vi "trace_toLVBuffer_spectrum.vi"(0 "reference":refnum<class "OSA.lvclass">, 2 "idx latest":bool, 3 "trace idx spectrum":u32, 5 "error in (no error)":errorcluster) -> (14 "duplicate reference":refnum<class "OSA.lvclass">, 16 "trace length":u32, 19 "error out":errorcluster)   [LabVIEW 2010, in "OSA.lvclass"]
doc: "Reads data from trace buffer and updates labview allocated buffer interferogram Y array, X is equidistant and only x min and max are retrieved. \n\nX: optical path length (cm)\nY: ADC value"
uses:
  OSA.lvclass
  typeDef/trace_properties_ui.ctl
  typeDef/trace_properties_double.ctl
  typeDef/acq_dataType.ctl
  typeDef/xVal_option.ctl
  FTSLib.dll
  OSA20X_misc.lvlib
panel:
  in  "property double":T1=enum."x_max"
  in  "property":T2=enum."interferogramProperty"
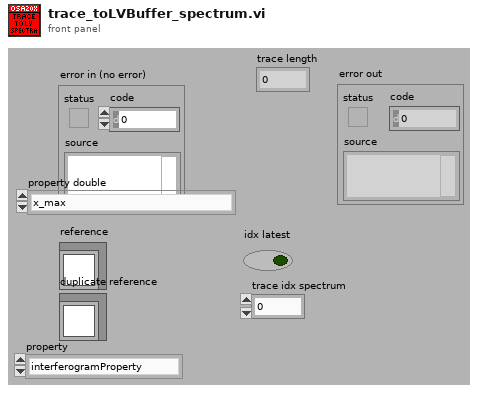
[diagram p1: front panel]
types:
  T1 = typedef "OSA.lvclass/trace_properties_double.ctl" = enum16{"x_minWnr", "x_maxWnr", "x_min", "x_max", "y_min", "y_max", "resolution", "referenceWavelength_nm_vac", "samplingDistance_cm_vac", "zeroFillFactor", "air_temp", "air_press", "air_relHum", "minOPD_cm", "maxOPD_cm", "interferogramOffset", "apodizationPowerCompensation", "integrationTime_ms", "gainLevel", "all_doubleProperties"}
  T2 = typedef "OSA.lvclass/trace_properties_ui.ctl" = enum16{"length", "type", "acquisitionMode", "xValueFormat", "date", "time", "averageNum", "smoothType", "igramSmoothType", "phaseCorrection", "apodisation", "__allocatedLengthI", "__allocatedLengthx", "adcBits", "sensitivityMode", "resolutionMode", "rollingAverage", "samplesPerReference", "air_measureOption", "interferogramProperty", "all_uiProperties"}
  T3 = typedef "OSA.lvclass/acq_dataType.ctl" = enum16{"none", "interferogram", "spectrum"}
  T4 = enum16{"get", "init", "set interferogram", "set spectrum", "cleanUp"}
  T5 = typedef "OSA.lvclass/xVal_option.ctl" = enum16{"MIN_MAX", "ARRAY"}
  T6 = typedef "OSA.lvclass/ObjectAttributes.ctl" = cluster{"Stop":bool, "dataType":T3, "spectrometerIdx":u16, "buffer size interferogram":i32, "interferogram":cluster{"new":bool, "plot_x_ min":sgl, "plot_x_max":sgl, "plot_y_min":sgl, "plot_y_max":sgl, "Graph Intrfrgrm":T7, "timeStamp":u32, "signal (%)":dbl, "traces":cluster{"idx":u32, "broadBand":bool, "monoChromatic":bool, "peakToPeakSignal":dbl, "peakToPeakPos":dbl}[], "traces idx last":i32}, "spectrum":cluster{"new":bool, "plot_x_min":sgl, "plot_x_max":sgl, "plot_unit_x":T8, "plot_unit_y":T9, "plot_y_min":sgl, "plot_y_max":sgl, "Graph Spectrum":T7, "timeStamp":u32, "X_VAL_OPTIONS":enum16{"MIN_MAX", "ARRAY"}, "traces":cluster{"idx":u32}[], "traces idx last":i32}, "Thorlabs_OSA_64.lvclass:queue_action.ctlqueue ref":refnum<queue>, "action":T10, "plot zoom step":dbl, "buffer semaphore":T11, "acq stopped":bool, "dataType active":T3, "temperature (degr C)":sgl, "pressure (hPa)":sgl, "rel humidity (%)":sgl, "settings":cluster{"resolution":T12, "sensitivity":T13, "Average":bool, "average nr":u32, "apodisation":T14, "acq delay (ms)":u32, "airMesure":T15, "wmtr on":bool, "intfgrm_smooth_width":u16, "intfgrm_smooth_nrOfPasses":u16, "intfgrm_smooth":T16, "phaseCorrection":T17, "zeroFill":u8, "spectr_smooth":T16, "spectr_smooth_width":u16, "spectr_smooth_nrOfPasses":u16, "resolution (/cm)":sgl, "REF wavelength, (nm)":dbl, "gain_idx":u16, "gainAuto":bool, "gain_relative":dbl, "PD sensitivity mode":T18, "PD senseMode implemented":bool, "SensorTemperature implemented":bool, "SensorPressure implemented":bool, "SensorHumidity implemented":bool}, "peaks position":sgl[], "peaks width":sgl[], "peaks height":sgl[], "peaks max nr":u32, "peaks latest nr":i32, "peaks new":bool, "power":dbl, "power new":bool, "path":string, "wavelength (WNr)":dbl, "wavelength new":bool, "buffer size spectrum":i32, "status":string, "VI reference":refnum<vi>, "funcPointer":u64, "libraryPointer":u64, "singleAcquisition":bool, "coherenceLength (cm)":dbl, "coherenceLength new":bool, "spectrometer model":string, "spectrometer serial nr":string, "peaks thld left":sgl[], "peaks thld right":sgl[], "coherenceLength error (cm)":dbl, "ADC bits":u16, "peaks position centroid":sgl[], "peaks height centroid":sgl[], "OSA series":T19, "channel index spectra":u16, "channel index interferogram":u16}
  T7 = typedef "OSA.lvclass/graph_intensity.ctl" = refnum<vi>
  T8 = typedef "OSA.lvclass/spectrum_x_unit.ctl" = enum16{"wavenr/cm", "THz", "eV", "nm_air", "nm_vac"}
  T9 = typedef "OSA.lvclass/y_unit.ctl" = enum16{"ADC counts", "dBm pwr absolute", "dBm pwr density", "mW pwr absolute", "mW pwr density"}
  T10 = typedef "OSA.lvclass/queue_action.ctl" = enum16{"none", "stop", "GUI_plotInterferogram", "GUI_plotSpectrum", "GUI_plotInterferogramRescale", "GUI_plotSpectrumRescale", "GUI_plotInterferogramReset", "GUI_plotSpectrumReset", "GUI_plotInterferogramAutoScaleY", "GUI_plotSpectrumAutoScaleY", "GUI_plotInterferogramZoomOut", "GUI_plotSpectrumZoomOut", "GUI_plotInterferogramPane", "GUI_plotSpectrumPane", "GUI_plotInterferogramZoomMouse", "GUI_plotSpectrumZoomMouse", "ENVIRONMENT temperature", "ENVIRONMENT pressure", "MODE_resolution set", "MODE_resolution get", "MODE_sensitivity set", "MODE_sensitivity get", "MODE_PDTemperature set", "MODE_PDTemperature get", "REBOOT/RESET firmware", "ACQASYNC_acquireSingleSpectrum", "ACQASYNC_continuous start", "ACQASYNC_continuous stop\n", "ACQASYNC_get last interferogram", "ACQASYNC_get last spectrum", "ACQASYNC_get last waveNr", "ACQOPT_interferogram smoothing set", "ACQOPT_interferogram smoothing get", "ACQOPT_spectrum smoothing set", "ACQOPT_spectrum smoothing get", "ACQOPT_apodisation type set", "ACQOPT_apodisation type get", "ACQOPT_phase correction type set", "ACQOPT_phase correction type get", "ACQOPT_acqIntervall_set", "ACQOPT_acqIntervall_get", "ACQOPT_average spectrum set", "ACQOPT_average spectrum get", "ACQOPT_rolling average set", "ACQOPT_rolling average get", "ACQOPT_zero fill factor set", "ACQOPT_zero fill factor get", "ACQOPT_cycle counting set", "ACQOPT_cycle counting get", "ACQOPT_air measure option set", "ACQOPT_air measure option get", "ACQOPT_gainLevel auto get", "ACQOPT_gainLevel auto set", "ACQOPT_gainLevel get", "ACQOPT_gainLevel set", "ACQOPT_getAll", "INSTRUMENT_PROPERTY_range_WaveNr_min", "INSTRUMENT_PROPERTY_range_WaveNr_max", "INSTRUMENT_PROPERTY_reference_wavelength_cm^-1", "INSTRUMENT_PROPERTY_samplesPerRefPeriod", "INSTRUMENT_PROPERTY_resolution_waveNrPercm", "INSTRUMENT_PROPERTY_availableGainLevels", "INSTRUMENT_PROPERTY_status", "CONVERT", "ANALYSE_POWER", "ANALYSE_PEAKS", "ANALYSE_WAVELENGTH", "ANALYSE_SPECTRUM", "ANALYSE_INTERFEROGRAM", "ANALYSE_COHERENCE_LENGTH", "MATH", "MATH_power", "MATH_peaks", "FILE", "miscellaneous"}
  T11 = typedef "Semaphore RefNum" = refnum<k1>
  T12 = typedef "OSA.lvclass/resolution.ctl" = enum16{"low", "high"}
  T13 = typedef "OSA.lvclass/sensitivityMode.ctl" = enum16{"low", "low medium", "high medium", "high"}
  T14 = typedef "OSA.lvclass/apodisation.ctl" = enum16{"NONE", "NORTON_BEER_WEAK", "NORTON_BEER_MEDIUM", "NORTON_BEER_STRONG", "TRIANGULAR", "COSINE", "HANN", "HAMMING", "BLACKMANHARRIS3", "BLACKMANHARRIS4", "GAUSSIAN"}
  T15 = typedef "OSA.lvclass/airMeasure.ctl" = enum16{"TEMPERATURE", "PRESSURE"}
  T16 = typedef "OSA.lvclass/smoothing.ctl" = enum16{"NONE", "BINOMIAL", "SAVITSKY_GOLAY", "FOURIER", "MOVING_AVERAGE", "GAUSSIAN"}
  T17 = typedef "OSA.lvclass/phaseCorrection.ctl" = enum16{"NONE", "MERTZ", "FORMAN", "MERTZ_FILE", "FORMAN_FILE", "FUTURE COMP."}
  T18 = typedef "OSA.lvclass/PDTemperatureMode.ctl" = enum16{"cool: better sensitivity/noise floor", "warm: extended wl range"}
  T19 = typedef "OSA.lvclass/OSA_series.ctl" = enum16{"OSA200", "OSA300", "UNKNOWN"}
  T20 = typedef "OSA20X.lvclass/xVal_option.ctl" = enum16{"MIN_MAX", "ARRAY"}
  T21 = cluster{"length":u32, "X min":sgl, "X max":sgl, "X_VAL_OPTIONS":T20}
  T22 = cluster{"idx":u32, "broadBand":bool, "monoChromatic":bool, "peakToPeakSignal":dbl, "peakToPeakPos":dbl}[]
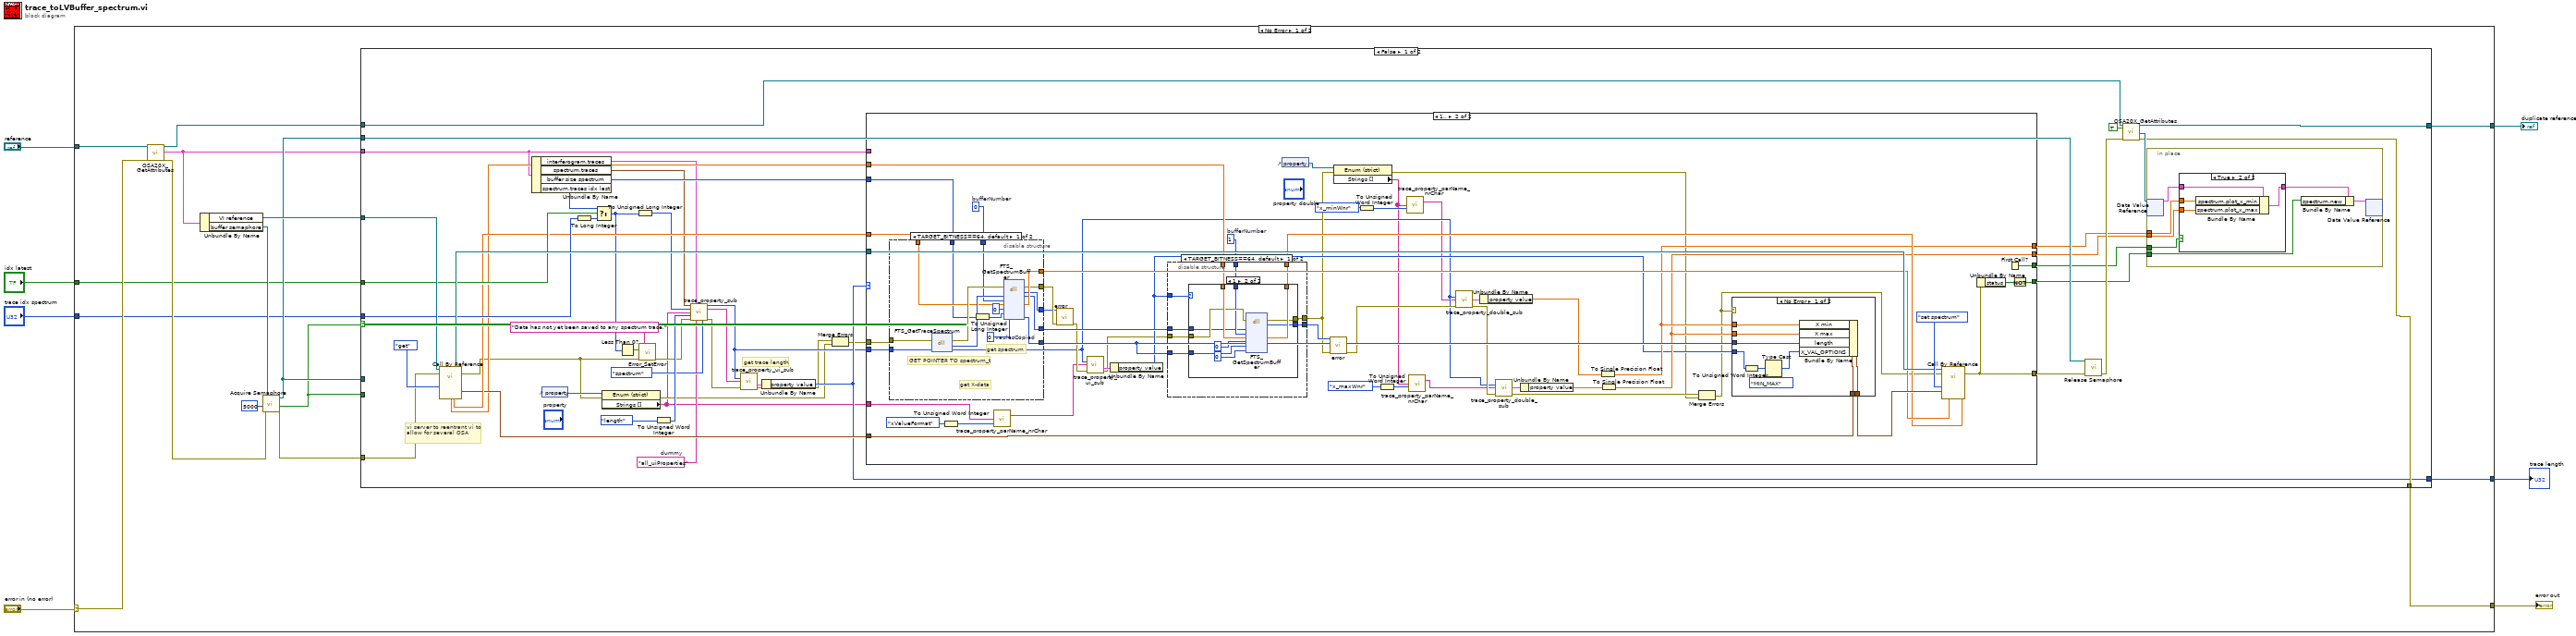
[diagram p0: block diagram]
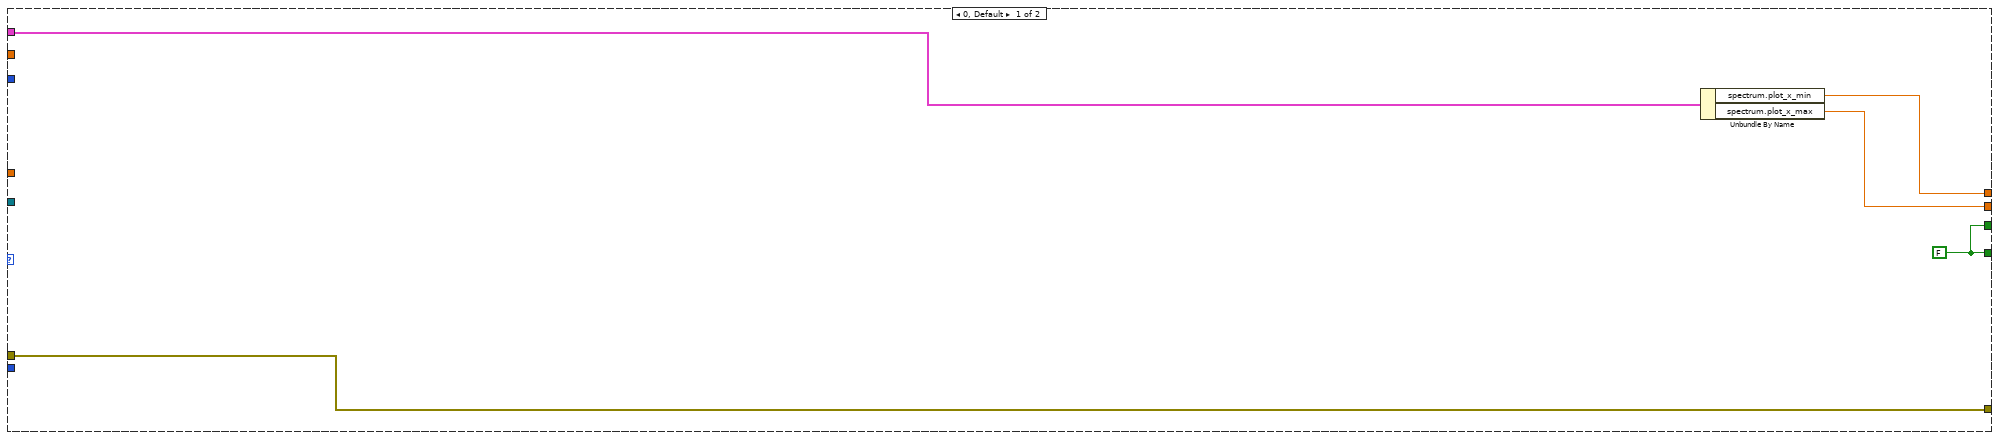
[diagram p2: hidden frame]
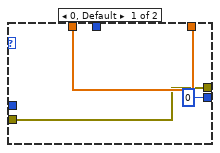
[diagram p3: hidden frame]
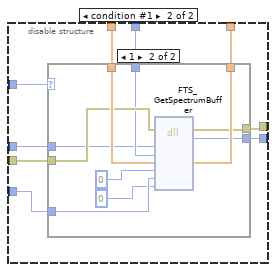
[diagram p4: hidden frame]
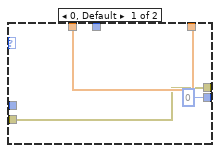
[diagram p5: hidden frame]
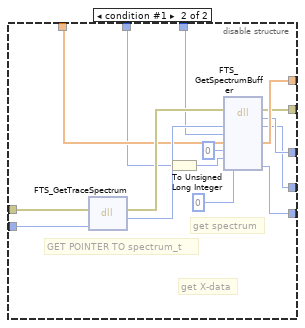
[diagram p7: hidden frame]
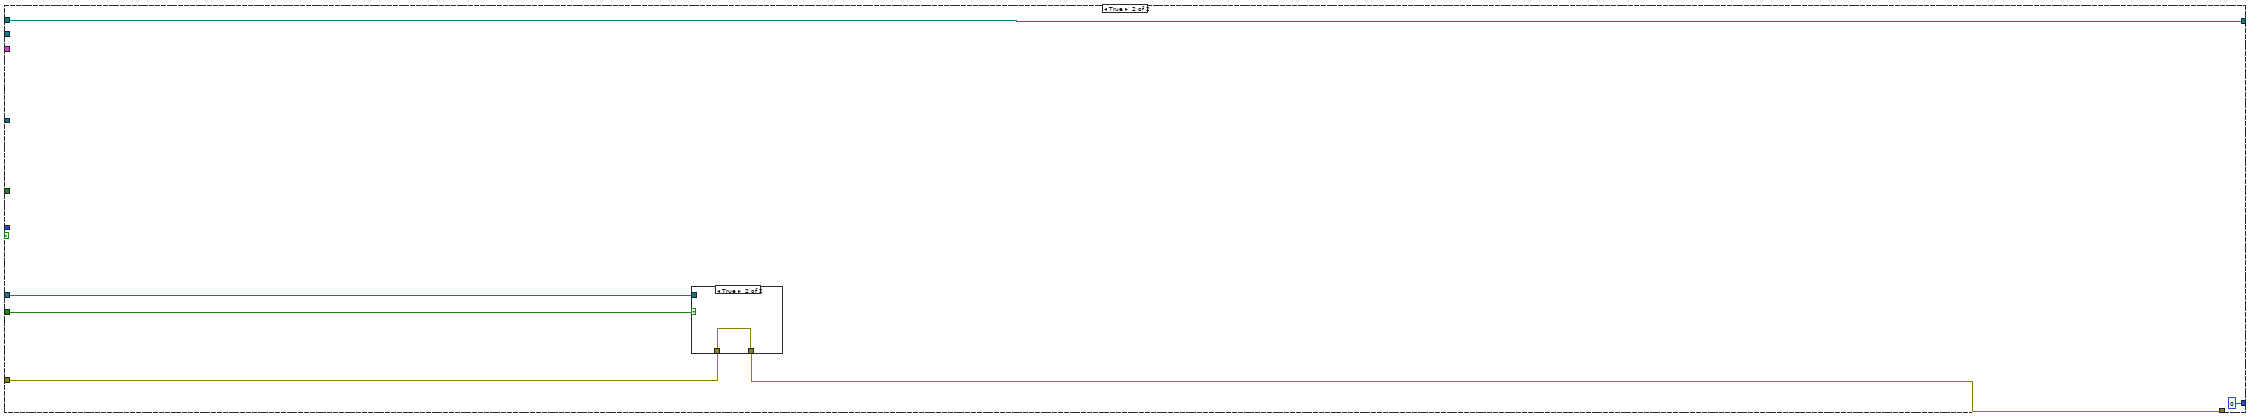
[diagram p9: hidden frame]
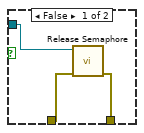
[diagram p10: hidden frame]
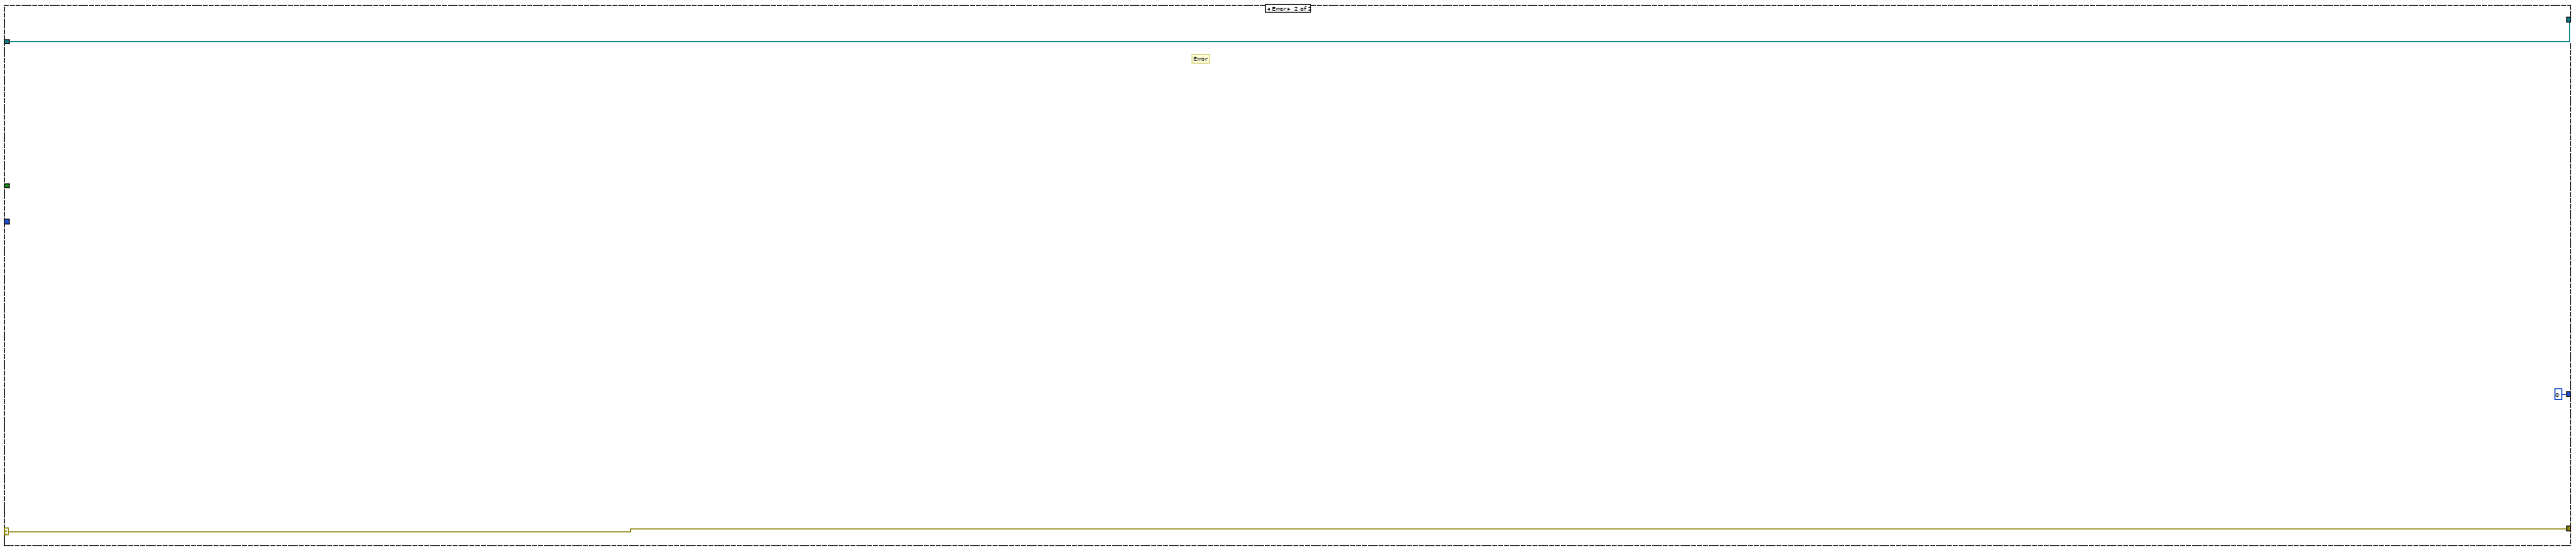
[diagram p11: hidden frame]
diagram:
  n1 = case shown="No Error" "error in (no error)" {
    selector: "error in (no error)" -> [w22 w234]
    tunnel: [w21 w234] -> w6
    tunnel: "reference" -> [w23 w233]
    tunnel: [w20 w233] -> w4
    tunnel: "idx latest" -> [w11 _]
    tunnel: "trace idx spectrum" -> [w10 _]
    tunnel: [w9 u32 0 ("property value")] -> w1
    frame No Error {
      n2 = call "OSA20X_GetAttributes.vi"("reference in"=w23, "error in (no error)"=w22) -> ("reference out"=w14:refnum<class "OSA.lvclass">, "Data"=w12:T6, "error out"=w18:errorcluster)  [unwired: 14 in, 1 out]
      n3 = Unbundle By Name(w12) -> ("VI reference"=w15:refnum<vi>, "buffer semaphore"=w19:T11)
      n4 = call <vilib>:"Acquire Semaphore.vi"("error in (no error)"=w18, "ms timeout (-1)"=5000, "semaphore"=w19) -> ("error out"=w16:errorcluster, "timed out"=w8:bool, "semaphore out"=w13:T11)  [unwired: 2 in]
      n5 = case shown="False" w8 {
        tunnel: w12 -> [w47 _]
        tunnel: w16 -> [w66 w224]
        tunnel: [w51 w223] -> w21
        tunnel: [w52 w227] -> w20
        tunnel: w13 -> [w68 _]
        tunnel: w15 -> [w65 _]
        tunnel: w14 -> [w25 w227]
        tunnel: w8 -> [_ w226]
        tunnel: w13 -> [_ w225]
        tunnel: w11 -> [w61 _]
        tunnel: w10 -> [w59 _]
        tunnel: [w30 u32 0 ("property value")] -> w9
        frame False {
          w32 = "all_uiProperties"  # dummy
          # "get trace length"
          # "vi server to reentrant vi to \nallow for several OSA"
          n6 = call-by-ref "?"(reference=w65, error in=w66, "action"=T4."get") -> (reference out=w64:refnum<vi>, error out=w43:errorcluster, "spectrum X"=w50:sgl[], "spectrum Y"=w54:sgl[], "spectrum property"=w53:T21)  [unwired: 14 in, 2 out]
          n7 = Unbundle By Name(w47) -> ("interferogram.traces"=w39:T22, "spectrum.traces"=w40:cluster{"idx":u32}[], "buffer size spectrum"=w55:i32, "spectrum.traces idx last"=w60:i32)
          n8 = control-ref of="property"() -> (w44:refnum<vi>)
          n9 = To Long Integer(number=w59) -> (32bit integer=w58:i32)
          n10 = Select(t=w60, s=w61, f=w58) -> (s? t:f=w41:i32)
          n11 = property class="Enum (strict)"(reference=w44, error in=w43) -> (error out=w27:errorcluster, "Strings []"=w24:string[])  [unwired: 1 out]
          n12 = Less Than 0?(x=w41) -> (x < 0?=w57:bool)
          n13 = To Unsigned Long Integer(number=w41) -> (unsigned 32bit integer=w38:u32)
          n14 = call "Error_SetError.vi"("error in"=w43, "status (true)"=w57, "source(\"\")"="Data has not yet been saved to any spectrum trace." ("source(\"\")")) -> ("error out"=w35:errorcluster)  [unwired: 4 in]
          n15 = To Unsigned Word Integer(number=trace_properties_ui."length" ("property")) -> (unsigned 16bit integer=w37:u16)
          n16 = call "trace_property_sub.vi"("traces_spectrum"=w40, "traces_interferogram"=w39, "trace idx"=w38, "Strings enum"=w24, "Value enum"=w37, "error in (no error)"=w35, "all string"=w32, "dataType"=acq_dataType."spectrum") -> ("global trace idx"=w29:u32, "parameter names"=w36:string[], "error out"=w34:errorcluster)  [unwired: 4 in, 1 out]
          n17 = call "trace_property_ui_sub.vi"("trace idx global"=w29, "properties ui"=w36, "error in (no error)"=w34) -> ("property"=w31:cluster{"property":string, "property value":u32}, "error out"=w28:errorcluster)  [unwired: 10 in, 1 out]
          n18 = Unbundle By Name(w31) -> ("property value"=w30:u32)
          n19 = Merge Errors(w28, w27) -> (w26:errorcluster)
          n20 = case shown="1.." w30 {
            tunnel: [w72 w105] -> w69
            tunnel: w64 -> [_ w124]
            tunnel: w55 -> [_ w123]
            tunnel: w54 -> [_ w122]
            tunnel: w53 -> [_ w121]
            tunnel: w29 -> [_ w88]
            tunnel: w26 -> [w72 w117]
            tunnel: w50 -> [_ w114]
            tunnel: [w74 w107] -> w49
            tunnel: [w73 w106] -> w48
            tunnel: w47 -> [w75 _]
            tunnel: [w71 w103] -> w46
            tunnel: [w71 w102] -> w45
            tunnel: w24 -> [_ w83]
            frame 0, Default {
              w71 = FALSE ("interferogram.new")
              n21 = Unbundle By Name(w75) -> ("spectrum.plot_x_min"=w74:sgl, "spectrum.plot_x_max"=w73:sgl)
            }
            frame 1.. {
              w112 = 1  # bufferNumber
              w119 = 0  # bufferNumber
              n22 = disable-structure shown="TARGET_BITNESS==64, default" {
                disable-tunnel: w117 -> [w193 w201]
                disable-tunnel: w88 -> [w194 w200]
                disable-tunnel: w122 -> [w190 w204]
                disable-tunnel: w123 -> [w188 w203]
                disable-tunnel: [w186 w199] -> w111
                disable-tunnel: [w185 w198] -> w118
                disable-tunnel: w119 -> [w183 w202]
                disable-tunnel: [w182 w197] -> w116
                disable-tunnel: [w181 w196] -> w115
                disable-tunnel: [w180 w195] -> w113
                frame condition #0 (active) {
                  w187 = u32 0  # vaulesCopied
                  # "get X-data"
                  # "get spectrum"
                  # "GET POINTER TO spectrum_t"
                  n23 = dll-call lib="FTSLib.dll" fn="FTS_GetTraceSpectrum"(error in=w193, "traceIdx"=w194) -> (error out=w192:errorcluster, "spectrum_t_pointer"=w191:u64)  [unwired: 3 in, 1 out]
                  n24 = To Unsigned Long Integer(number=w188) -> (unsigned 32bit integer=w184:u32)
                  n25 = dll-call lib="FTSLib.dll" fn="FTS_GetSpectrumBuffer"(error in=w192, "source"=w191, "bufferNumber"=w183, "destination"=w190, "startIndex"=u32 0, "length"=w184, "vaulesCopied"=w187) -> (error out=w182:errorcluster, "return type"=w181:i32, "source"=w180:u64, "destination"=w185:sgl[], "vaulesCopied"=w186:u32)  [unwired: 5 in, 1 out]
                }
                frame condition #1 {
                  # "get X-data"
                  # "get spectrum"
                  # "GET POINTER TO spectrum_t"
                  n26 = dll-call lib="FTSLib.dll" fn="FTS_GetTraceSpectrum"(error in=w201, "traceIdx"=w200) -> (error out=w209:errorcluster, "spectrum_t_pointer"=w208:u32)  [unwired: 3 in, 1 out]
                  n27 = To Unsigned Long Integer(number=w203) -> (unsigned 32bit integer=w205:u32)
                  n28 = dll-call lib="FTSLib.dll" fn="FTS_GetSpectrumBuffer"(error in=w209, "source"=w208, "bufferNumber"=w202, "destination"=w204, "startIndex"=u32 0, "length"=w205, "vaulesCopied"=u32 0) -> (error out=w197:errorcluster, "return type"=w196:i32, "source"=w195:u32, "destination"=w198:sgl[], "vaulesCopied"=w199:u32)  [unwired: 5 in, 1 out]
                }
              }
              n29 = To Unsigned Word Integer(number=trace_properties_ui."xValueFormat" ("property")) -> (unsigned 16bit integer=w82:u16)
              n30 = call "trace_property_parName_nrChar.vi"("Strings enum"=w83, "Value enum"=w82) -> ("parameter names"=w81:string[])  [unwired: 12 in, 1 out]
              n31 = call "error.vi"("result code"=w115, "error in (no error)"=w116) -> ("error out"=w100:errorcluster)  [unwired: 15 in, 2 out]
              n32 = call "trace_property_ui_sub.vi"("trace idx global"=w88, "properties ui"=w81, "error in (no error)"=w100) -> ("property"=w99:cluster{"property":string, "property value":u32}, "error out"=w97:errorcluster)  [unwired: 10 in, 1 out]
              n33 = Unbundle By Name(w99) -> ("property value"=w98:u32)
              n34 = disable-structure shown="TARGET_BITNESS==64, default" {
                disable-tunnel: w97 -> [w134 w151]
                disable-tunnel: w98 -> [w133 w150]
                disable-tunnel: w114 -> [w132 w153]
                disable-tunnel: w113 -> [w131 w149]
                disable-tunnel: w112 -> [w130 w148]
                disable-tunnel: w111 -> [w129 w156]
                disable-tunnel: [w128 w154] -> w96
                disable-tunnel: [w127 w155] -> w110
                disable-tunnel: [w126 w152] -> w109
                frame condition #0 (active) {
                  n35 = case shown="1" w133 {
                    tunnel: [w136 w139] -> w128
                    tunnel: w132 -> [w137 w146]
                    tunnel: w134 -> [w136 w145]
                    tunnel: [w137 w144] -> w126
                    tunnel: w129 -> [_ w143]
                    tunnel: w130 -> [_ w141]
                    tunnel: w131 -> [_ w140]
                    tunnel: [0 ("return type") w138] -> w127
                    frame 0, Default {
                    }
                    frame 1 {
                      n36 = dll-call lib="FTSLib.dll" fn="FTS_GetSpectrumBuffer"(error in=w145, "source"=w140, "bufferNumber"=w141, "destination"=w146, "startIndex"=u32 0, "length"=w143, "vaulesCopied"=u32 0) -> (error out=w139:errorcluster, "return type"=w138:i32, "destination"=w144:sgl[])  [unwired: 7 in, 1 out]
                    }
                  }
                }
                frame condition #1 {
                  n37 = case shown="1" w150 {
                    tunnel: [w158 w161] -> w154
                    tunnel: w153 -> [w159 w168]
                    tunnel: w151 -> [w158 w167]
                    tunnel: [w159 w166] -> w152
                    tunnel: w156 -> [_ w165]
                    tunnel: w148 -> [_ w163]
                    tunnel: w149 -> [_ w162]
                    tunnel: [0 ("return type") w160] -> w155
                    frame 0, Default {
                    }
                    frame 1 {
                      n38 = dll-call lib="FTSLib.dll" fn="FTS_GetSpectrumBuffer"(error in=w167, "source"=w162, "bufferNumber"=w163, "destination"=w168, "startIndex"=u32 0, "length"=w165, "vaulesCopied"=u32 0) -> (error out=w161:errorcluster, "return type"=w160:i32, "destination"=w166:sgl[])  [unwired: 7 in, 1 out]
                    }
                  }
                }
              }
              n39 = control-ref of="property double"() -> (w95:refnum<vi>)
              n40 = call "error.vi"("result code"=w110, "error in (no error)"=w96) -> ("error out"=w93:errorcluster)  [unwired: 15 in, 2 out]
              n41 = property class="Enum (strict)"(reference=w95, error in=w96) -> (error out=w85:errorcluster, "Strings []"=w77:string[])  [unwired: 1 out]
              n42 = To Unsigned Word Integer(number=trace_properties_double."x_minWnr" ("property")) -> (unsigned 16bit integer=w80:u16)
              n43 = To Unsigned Word Integer(number=trace_properties_double."x_maxWnr" ("property")) -> (unsigned 16bit integer=w78:u16)
              n44 = call "trace_property_parName_nrChar.vi"("Strings enum"=w77, "Value enum"=w80) -> ("parameter names"=w79:string[])  [unwired: 12 in, 1 out]
              n45 = call "trace_property_parName_nrChar.vi"("Strings enum"=w77, "Value enum"=w78) -> ("parameter names"=w76:string[])  [unwired: 12 in, 1 out]
              n46 = call "trace_property_double_sub.vi"("trace idx global"=w88, "properties ui"=w79, "error in (no error)"=w93) -> ("property"=w92:cluster{"property":string, "property value":dbl}, "error out"=w89:errorcluster)  [unwired: 10 in, 1 out]
              n47 = Unbundle By Name(w92) -> ("property value"=w91:dbl)
              n48 = call "trace_property_double_sub.vi"("trace idx global"=w88, "properties ui"=w76, "error in (no error)"=w89) -> ("property"=w87:cluster{"property":string, "property value":dbl}, "error out"=w86:errorcluster)  [unwired: 10 in, 1 out]
              n49 = Unbundle By Name(w87) -> ("property value"=w108:dbl)
              n50 = To Single Precision Float(number=w91) -> (single precision float=w107:sgl)
              n51 = To Single Precision Float(number=w108) -> (single precision float=w106:sgl)
              n52 = Merge Errors(w86, w85) -> (w84:errorcluster)
              n53 = case shown="No Error" w84 {
                tunnel: w121 -> [w178 w179]
                tunnel: w111 -> [w177 _]
                tunnel: [w176 w179] -> w120
                tunnel: w98 -> [w174 _]
                tunnel: w106 -> [w171 _]
                tunnel: w107 -> [w170 _]
                frame No Error {
                  n54 = To Unsigned Word Integer(number=w174) -> (unsigned 16bit integer=w173:u16)
                  n55 = Type Cast(type=xVal_option."MIN_MAX" ("X_VAL_OPTIONS"), x=w173) -> (*(type *) &x=w172:T5)
                  n56 = Bundle By Name(cluster=w178, "X min"=w170, "X max"=w171, "length"=w177, "X_VAL_OPTIONS"=w172) -> (w176:T21)
                }
                frame Error {
                }
              }
              n57 = call-by-ref "?"(reference=w124, error in=w84, "action"=T4."set spectrum", "spectrum prop set"=w120, "spectrum set Y"=w118, "spectrum set X"=w109) -> (error out=w105:errorcluster)  [unwired: 11 in, 6 out]
              n58 = Unbundle By Name(w105) -> ("status"=w104:bool)
              n59 = First Call?() -> (First Call?: T/F=w102:bool)
              n60 = Not(x=w104) -> (.not. x?=w103:bool)
            }
          }
          n61 = call <vilib>:"Release Semaphore.vi"("error in (no error)"=w69, "semaphore"=w68) -> ("error out"=w70:errorcluster)  [unwired: 4 in, 1 out]
          n62 = call "OSA20X_GetAttributes.vi"("reference in"=w25, "OnlyGetDvrReference(False)"=TRUE, "error in (no error)"=w70) -> ("reference out"=w52:refnum<class "OSA.lvclass">, "DataRef"=w62:refnum<data-value>, "error out"=w51:errorcluster)  [unwired: 13 in, 1 out]
          n63 = in-place {
            in-place-border: w45 -> [w216]
            in-place-border: w49 -> [w214]
            in-place-border: w48 -> [w213]
            in-place-border: w46 -> [w211]
            n64 = in-place-dvr #1(w62) -> (w215:T6)  [unwired: 1 out]
            n65 = case shown="True" w216 {
              tunnel: w215 -> [w217 w221]
              tunnel: [w217 w220] -> w212
              tunnel: w214 -> [_ w219]
              tunnel: w213 -> [_ w218]
              frame False {
              }
              frame True {
                n66 = Bundle By Name(cluster=w221, "spectrum.plot_x_min"=w219, "spectrum.plot_x_max"=w218) -> (w220:T6)
              }
            }
            n67 = Bundle By Name(cluster=w212, "spectrum.new"=w211) -> (w210:T6)
            n68 = in-place-dvr #1(w210) -> ()  [unwired: 2 out]
          }
        }
        frame True {
          n69 = case shown="True" w226 {
            tunnel: w225 -> [w230 _]
            tunnel: w224 -> [w229 w231]
            tunnel: [w228 w231] -> w223
            frame False {
              n70 = call <vilib>:"Release Semaphore.vi"("error in (no error)"=w229, "semaphore"=w230) -> ("error out"=w228:errorcluster)  [unwired: 4 in, 1 out]
            }
            frame True {
            }
          }
        }
      }
    }
    frame Error {
      # "Error"
    }
  }
  "error out" <- w6
  "duplicate reference" <- w4
  "trace length" <- w1
